vi "[GV]_EKF State Vector.vi"() -> ()   [LabVIEW 2016]
panel:
  out "EKF State Vector":dbl[][](array[numeric])
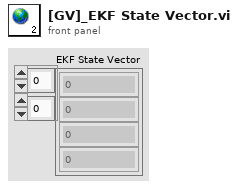
[diagram p1: front panel]
diagram:
